vi "Creator.vi"(9 "Is Priority":bool, 10 "Msg":refnum<class "Msg.lvclass">, 11 "Base Actor in":refnum<class "Base Actor.lvclass">) -> (3 "Base Actor out":refnum<class "Base Actor.lvclass">)   [LabVIEW 2020, in "jettl.lvlib" / "Actor.lvlib" / "Base Actor.lvclass"]
uses:
  Base Actor.lvclass
  Sender/Relation.ctl
  Sender/Sender.lvlib
  Msg/Msg.lvclass
  Error/Error.lvlib
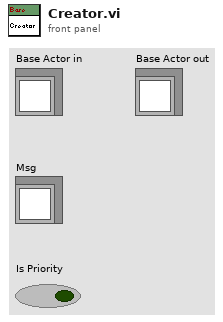
[diagram p1: front panel]
types:
  T1 = typedef "jettl.lvlib/Actor.lvlib/Implemented Msgs.ctl" = set{refnum<class "Msg.lvclass">}
  T2 = typedef "jettl.lvlib/Sender.lvlib/Relation.ctl" = enum16{"Self", "Creator", "Created"}
  T3 = typedef "jettl.lvlib/Actor.lvlib/Attributes.ctl" = cluster{"Alias":string, "Address":refnum<user-event>, "Implemented Msgs":T1, "Path":path}
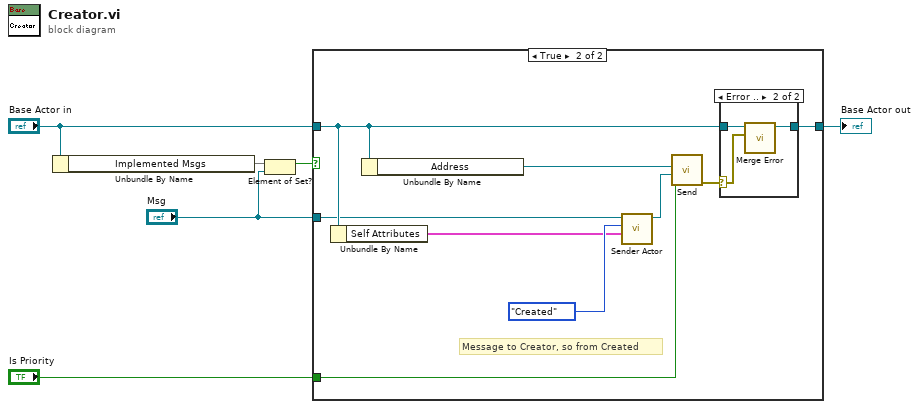
[diagram p0: block diagram]
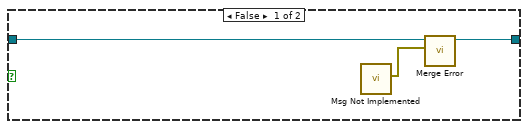
[diagram p2: hidden frame]
diagram:
  n1 = Unbundle By Name("Base Actor in") -> ("Implemented Msgs"=w3:T1)
  n2 = Element of Set?(10:"Msg", 11:w3) -> (3:w1:bool)
  n3 = case shown="True" w1 {
    tunnel: "Is Priority" -> [_ w17]
    tunnel: [w7 w16] -> w5
    tunnel: "Base Actor in" -> [w8 w14]
    tunnel: "Msg" -> [_ w12]
    frame False {
      n4 = call "Msg Not Implemented.vi"() -> ("Error"=w9:errorcluster)  [unwired: 11 in]
      n5 = call-dynamic "Merge Error.vi"("Error"=w9, "Base Actor in"=w8) -> ("Base Actor out"=w7:refnum<class "Base Actor.lvclass">)  [unwired: 9 in]
    }
    frame True {
      # "Message to Creator, so from Created"
      n6 = Unbundle By Name(w14) -> ("Self Attributes"=w10:T3)
      n7 = Unbundle By Name(w14) -> ("Address"=w15:refnum<user-event>)
      n8 = call "Sender Actor.vi"("Self Attributes"=w10, "Relation"=Relation."Created", "Msg in"=w12) -> ("Msg out"=w13:refnum<class "Msg.lvclass">)  [unwired: 8 in]
      n9 = call "Send.vi"("Is Priority"=w17, "Msg"=w13, "Address"=w15) -> ("error out"=w18:errorcluster)  [unwired: 8 in]
      n10 = case shown="Error .." w18 {
        selector: w18 -> [_ w20]
        tunnel: [w19 w22] -> w16
        tunnel: w14 -> [w19 w21]
        frame No Error {
        }
        frame Error {
          n11 = call-dynamic "Merge Error.vi"("Error"=w20, "Base Actor in"=w21) -> ("Base Actor out"=w22:refnum<class "Base Actor.lvclass">)  [unwired: 9 in]
        }
      }
    }
  }
  "Base Actor out" <- w5
